vi "Framework.Initialize Engine Pointer.vi"(8 "error in (no error)":errorcluster, 10 "Engine Pointer":refnum<class "Memory.Pointer.lvclass">, 11 "Framework in":refnum<class "Framework.lvclass">) -> (0 "error out":errorcluster, 3 "Framework out":refnum<class "Framework.lvclass">)   [LabVIEW 2017, in "DSF Core.lvlib" / "Framework.lvclass"]
uses:
  Framework.lvclass
  <vilib>/NI/Memory Manager/Classes/Pointer/Memory.Pointer.lvclass
  Framework.lvclass/Framework.ctl
  Framework.Get Engine Pointer.vi
  Plugin/Plugin.Offset Inline Buffers.vi
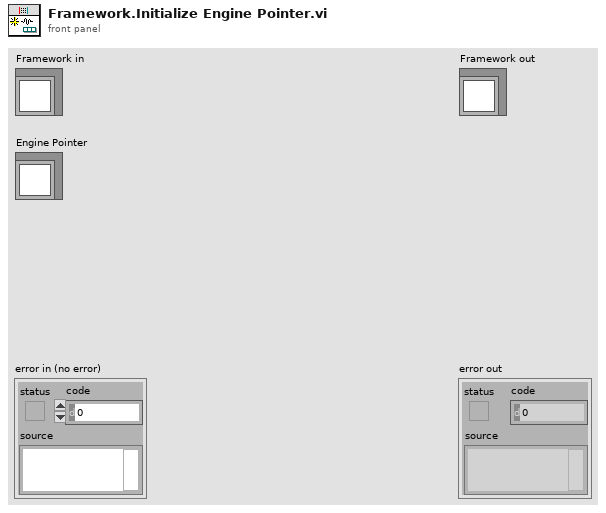
[diagram p1: front panel]
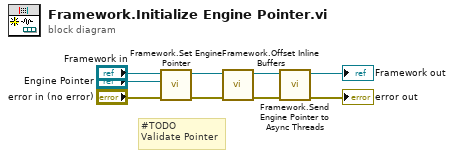
[diagram p0: block diagram]
diagram:
  # "#TODO\nValidate Pointer"
  n1 = call "Framework.Set Engine Pointer.vi"("Engine Pointer"="Engine Pointer", "Framework in"="Framework in") -> ("Framework out"=w7:refnum<class "Framework.lvclass">)  [unwired: 9 in]
  n2 = call "Framework.Offset Inline Buffers.vi"("error in (no error)"="error in (no error)", "Framework in"=w7) -> ("error out"=w4:errorcluster, "Framework out"=w5:refnum<class "Framework.lvclass">)  [unwired: 8 in]
  n3 = call "Framework.Send Engine Pointer to Async Threads.vi"("error in (no error)"=w4, "Framework in"=w5) -> ("error out"=→"error out":errorcluster, "Framework out"=→"Framework out":refnum<class "Framework.lvclass">)  [unwired: 8 in]
